vi "Generate Results.vi"(8 "error in (no error)":errorcluster, 10 "Storage":refnum<class "Test Event Storage.lvclass">, 11 "Basic Test Manager in":refnum<class "Basic Test Manager.lvclass">) -> (0 "error out":errorcluster, 2 "Test Result":refnum<class "Test Result.lvclass">, 3 "Basic Test Manager out":refnum<class "Basic Test Manager.lvclass">)   [LabVIEW 2009, in "Caraya.lvlib" / "Basic Test Manager.lvclass"]
uses:
  Basic Test Manager.lvclass
  Test Event Storage/Test Event Storage.lvclass
  Test Result/Test Result.lvclass
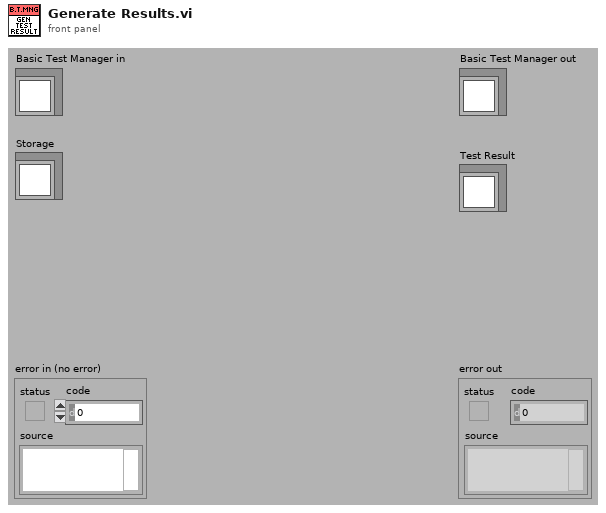
[diagram p1: front panel]
types:
  T1 = typedef "Caraya.lvlib/Test Event Storage.lvclass/Test Node.ctl" = cluster{"Test Registration":T2, "Defined":bool, "Passed":bool}
  T2 = typedef "Caraya.lvlib/Basic Test Manager.lvclass/Test Registration Data.ctl" = cluster{"Name":string, "Call Chain":string[], "Time Stamp":timestamp}
  T3 = typedef "Caraya.lvlib/Basic Test Manager.lvclass/Assert Event Data.ctl" = cluster{"Name":string, "Passed":bool, "Call Chain":string[], "Test Error":errorcluster, "Time Stamp":timestamp}
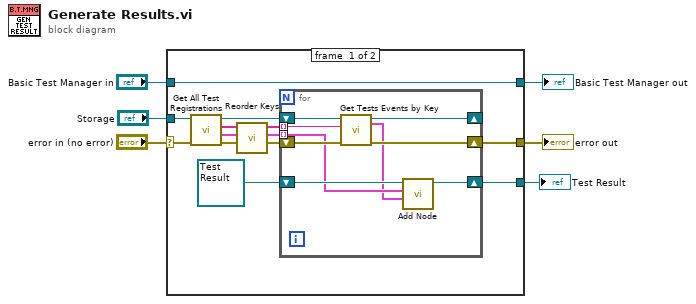
[diagram p0: block diagram]
diagram:
  n1 = case shown="No Error" "error in (no error)" {
    selector: "error in (no error)" -> [w16 w29]
    tunnel: [w14 w29] -> w5
    tunnel: [w11 w28] -> w3
    tunnel: "Basic Test Manager in" -> [w11 w28]
    tunnel: "Storage" -> [w18 _]
    tunnel: [w13 _] -> w1
    frame #0 {
      n2 = call-dynamic "Get All Test Registrations.vi"("error in (no error)"=w16, "Test Event Storage in"=w18) -> ("error out"=w15:errorcluster, "Test Registrations"=w8:T1[], "Keys"=w10:string[], "Test Event Storage out"=w17:refnum<class "Test Event Storage.lvclass">)  [unwired: 5 in, 1 out]
      n3 = call "Reorder Keys.vi"("Test Registrations in"=w8, "Keys in"=w10) -> ("Test Registrations out"=w7:T1[], "Keys out"=w9:string[])  [unwired: 8 in]
      n4 = for {
        tunnel: w7 -> [w21] mode=indexing
        tunnel: w9 -> [w26] mode=indexing
        shift-right: [w19] -> w13
        shift-left: refnum<class "Test Result.lvclass"> refnum ("Caraya.lvlib:Test Result.lvclass") -> [w22]
        shift-right: [w25] -> _
        shift-left: w17 -> [w27]
        shift-right: [w23] -> w14
        shift-left: w15 -> [w24]
        n5 = call "Get Tests Events by Key.vi"("error in (no error)"=w24, "Key"=w26, "Test Event Storage in"=w27) -> ("error out"=w23:errorcluster, "Test Events"=w20:T3[], "Test Event Storage out"=w25:refnum<class "Test Event Storage.lvclass">)  [unwired: 6 in]
        n6 = call "Add Node.vi"("Test Events"=w20, "Test Node"=w21, "Test Result in"=w22) -> ("Test Result out"=w19:refnum<class "Test Result.lvclass">)  [unwired: 7 in, 1 out]
      }
    }
    frame #1 {
    }
  }
  "error out" <- w5
  "Basic Test Manager out" <- w3
  "Test Result" <- w1
